vi "Read GUI Settings (SubVI).vi"(11 "File Path":path=path "C:/MWT/Config.ini") -> (3 "GUI Parameters":T1={"Image Width"=3072, "Image Height"=3072, "Pixel Intensity Low"=25, "Pixel Intensity High"=135, "Box Side Low"=6, "Box Side High"=200, "Box W+L Low"=12, "Box W+L High"=200, "Area Low"=12, "Area High"=200, "BG SUB TH"=200, "N Spine Points"=11.0, "Min Contour Points"=127, "Pixel Resolution (um/Pixel)"=40.69, "Gamma"=0.2} {"Gamma" format="%#_13g"; "Pixel Resolution (um/Pixel)" format="%#_13g"})   [LabVIEW 2020]
uses:
  Controls (HOST)/GUI Param.ctl
  Controls (HOST)/GUI Param List.ctl
  <vilib>/Utility/config.llb/Read Key (U32).vi
  <vilib>/Utility/config.llb/Write Key (U32).vi
  <vilib>/Utility/config.llb/Read Key (I32).vi
  <vilib>/Utility/config.llb/Write Key (I32).vi
  <vilib>/Utility/config.llb/Read Key (Double).vi
  <vilib>/Utility/config.llb/Write Key (Double).vi
  <vilib>/Utility/config.llb/NI_LVConfig.lvlib
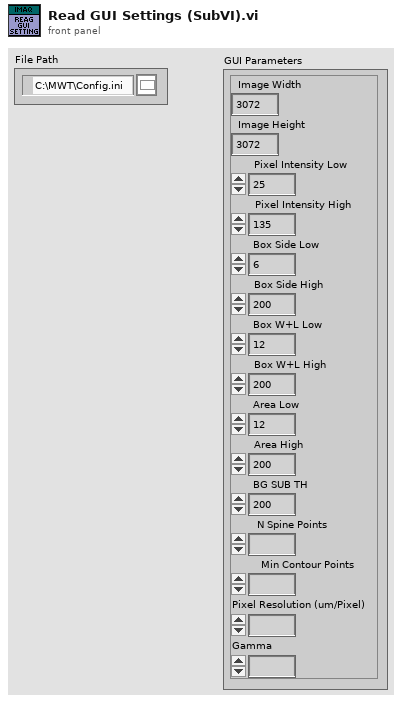
[diagram p1: front panel]
types:
  T1 = typedef "GUI Param.ctl" = cluster{"Image Width":u16, "Image Height":u16, "Pixel Intensity Low":u8, "Pixel Intensity High":u8, "Box Side Low":u32, "Box Side High":u32, "Box W+L Low":u32, "Box W+L High":u32, "Area Low":u32, "Area High":u32, "BG SUB TH":i16, "N Spine Points":fxp<+,8,8>, "Min Contour Points":u16, "Pixel Resolution (um/Pixel)":dbl, "Gamma":dbl}
  T2 = typedef "GUI Param List.ctl" = enum16{"None", "Image Height", "Image Width", "Pixel Intensity Low", "Pixel Intensity High", "Box Side Low", "Box Side High", "Box W+L Low", "Box W+L High", "Area Low", "Area High", "BG Sub Threshold", "N Spine Points", "Min Contour Points", "Pixel Resolution", "Gamma"}
  T3 = typedef "NI_LVConfig.lvlib/Config Data RefNum.ctl" = refnum<k1>
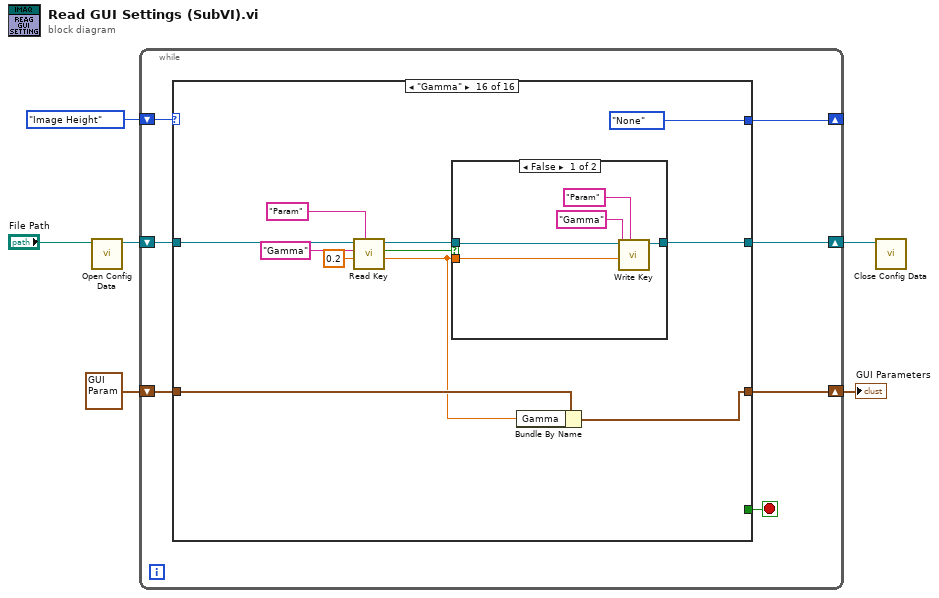
[diagram p0: block diagram]
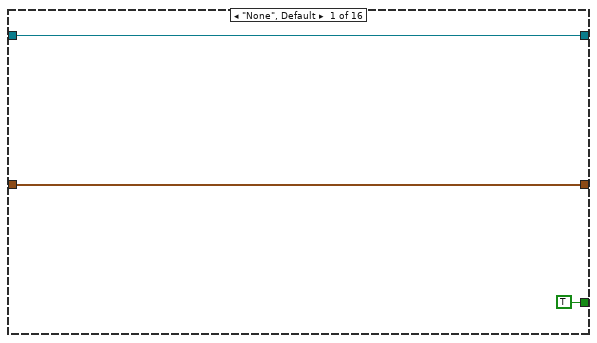
[diagram p2: hidden frame]
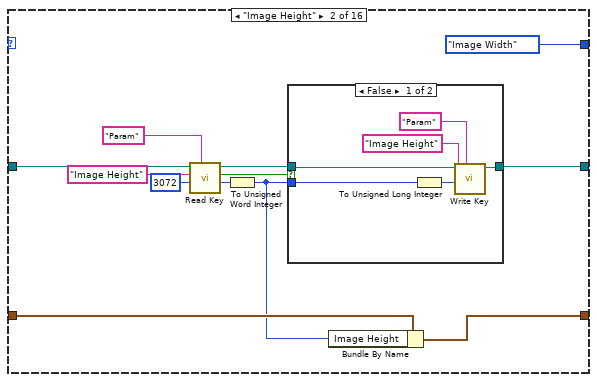
[diagram p3: hidden frame]
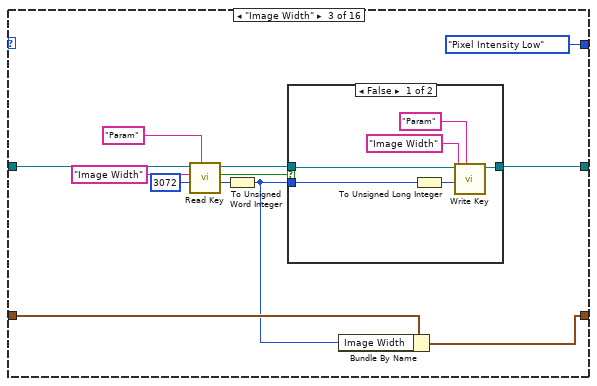
[diagram p5: hidden frame]
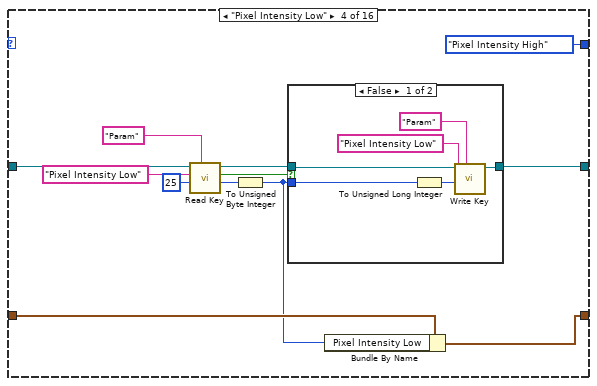
[diagram p7: hidden frame]
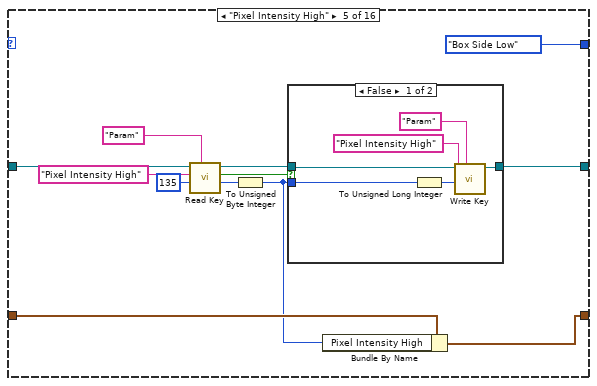
[diagram p9: hidden frame]
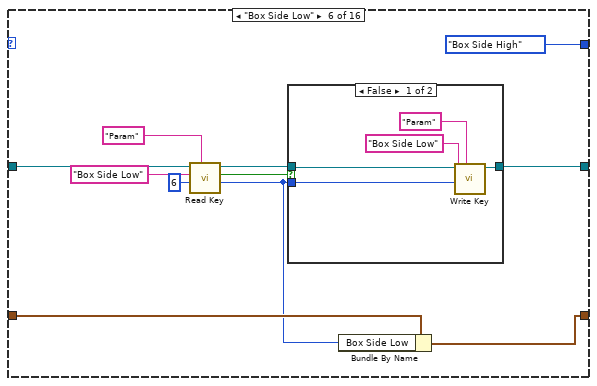
[diagram p11: hidden frame]
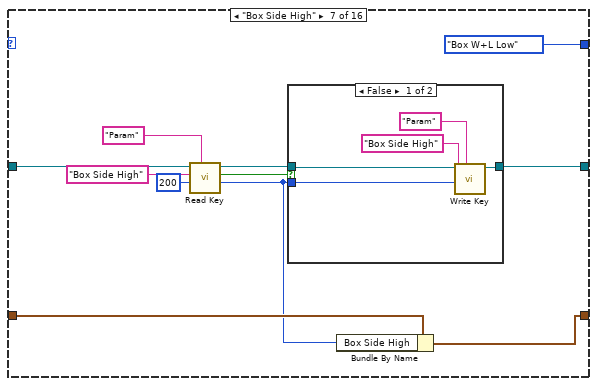
[diagram p13: hidden frame]
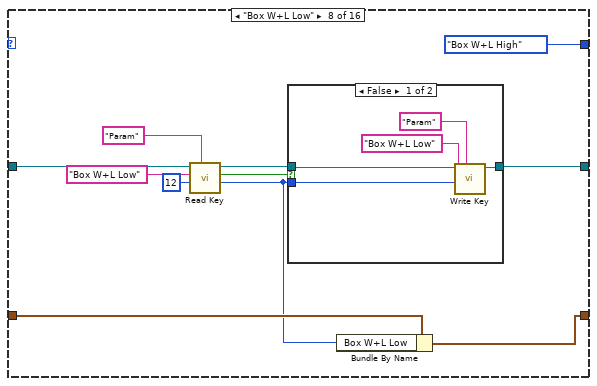
[diagram p15: hidden frame]
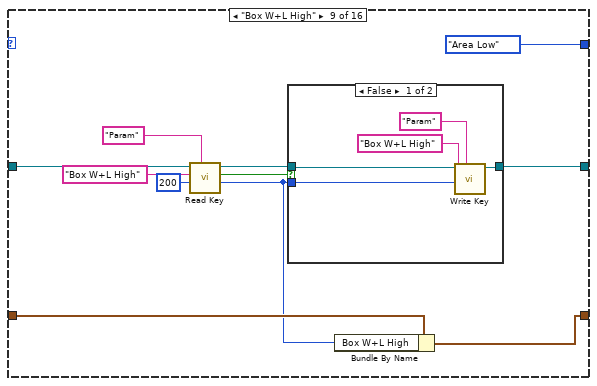
[diagram p17: hidden frame]
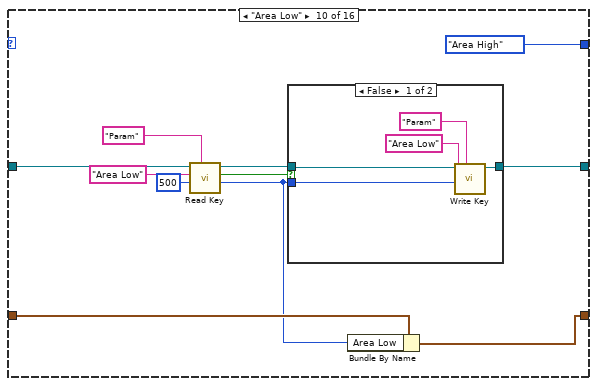
[diagram p19: hidden frame]
diagram:
  n1 = call <vilib>:"Open Config Data.vi"("configuration file path"="File Path") -> ("refnum"=w6:T3)  [unwired: 8 in, 2 out]
  n2 = while {
    shift-right: [w12] -> w4
    shift-left: w6 -> [w13]
    shift-right: [w9] -> _
    shift-left: GUI_Param_List."Image Height" -> [w11]
    shift-right: [w7] -> w1
    shift-left: T1 {"Image Width"=3072, "Image Height"=3072, "Pixel Intensity Low"=25, "Pixel Intensity High"=135, "Box Side Low"=6, "Box Side High"=200, "Box W+L Low"=12, "Box W+L High"=200, "Area Low"=12, "Area High"=200, "BG SUB TH"=200, "N Spine Points"=11.0, "Min Contour Points"=200, "Pixel Resolution (um/Pixel)"=40.69, "Gamma"=0.2} -> [w8]
    stop <- w10 stop-if-true
    n3 = case shown="\"Gamma\"" w11 {
      tunnel: w13 -> [w16 w24 w43 w63 w82 w100 w117 w134 w151 w168 w185 w203 w221 w239 w256 w273]
      tunnel: [w16 w21 w40 w60 w79 w97 w114 w131 w148 w165 w182 w200 w218 w236 w253 w270] -> w12
      tunnel: [TRUE _ _ _ _ _ _ _ _ _ _ _ _ _ _ _] -> w10
      tunnel: [_ GUI_Param_List."Image Width" GUI_Param_List."Pixel Intensity Low" GUI_Param_List."Pixel Intensity High" GUI_Param_List."Box Side Low" GUI_Param_List."Box Side High" GUI_Param_List."Box W+L Low" GUI_Param_List."Box W+L High" GUI_Param_List."Area Low" GUI_Param_List."Area High" GUI_Param_List."BG Sub Threshold" GUI_Param_List."N Spine Points" GUI_Param_List."Min Contour Points" GUI_Param_List."Pixel Resolution" GUI_Param_List."Gamma" GUI_Param_List."None"] -> w9
      tunnel: w8 -> [w14 w19 w38 w58 w77 w95 w112 w129 w146 w163 w180 w198 w216 w234 w251 w268]
      tunnel: [w14 w18 w37 w57 w76 w94 w111 w128 w145 w162 w179 w197 w215 w233 w250 w267] -> w7
      frame "None", Default {
      }
      frame "Image Height" {
        n4 = call-poly <vilib>:"Read Key.vi"("section"="Param", "default value"=u32 3072, "key"="Image Height" ("section"), "refnum"=w24) -> ("value"=w28:u32, "found?"=w23:bool, "refnum out"=w22:T3)  [unwired: 4 in, 1 out]
        n5 = To Unsigned Word Integer(number=w28) -> (unsigned 16bit integer=w17:u16)
        n6 = case shown="False" w23 {
          tunnel: w22 -> [w31 w35]
          tunnel: [w30 w35] -> w21
          tunnel: w17 -> [w29 _]
          frame False {
            n7 = To Unsigned Long Integer(number=w29) -> (unsigned 32bit integer=w33:u32)
            n8 = call-poly <vilib>:"Write Key.vi"("section"="Param", "value"=w33, "key"="Image Height" ("section"), "refnum"=w31) -> ("refnum out"=w30:T3)  [unwired: 5 in, 2 out]
          }
          frame True {
          }
        }
        n9 = Bundle By Name(cluster=w19, "Image Height"=w17) -> (w18:T1)
      }
      frame "Image Width" {
        n10 = call-poly <vilib>:"Read Key.vi"("section"="Param", "default value"=u32 3072, "key"="Image Width" ("section"), "refnum"=w43) -> ("value"=w47:u32, "found?"=w42:bool, "refnum out"=w41:T3)  [unwired: 4 in, 1 out]
        n11 = To Unsigned Word Integer(number=w47) -> (unsigned 16bit integer=w36:u16)
        n12 = case shown="False" w42 {
          tunnel: w41 -> [w50 w54]
          tunnel: [w49 w54] -> w40
          tunnel: w36 -> [w48 _]
          frame False {
            n13 = To Unsigned Long Integer(number=w48) -> (unsigned 32bit integer=w52:u32)
            n14 = call-poly <vilib>:"Write Key.vi"("section"="Param", "value"=w52, "key"="Image Width" ("section"), "refnum"=w50) -> ("refnum out"=w49:T3)  [unwired: 5 in, 2 out]
          }
          frame True {
          }
        }
        n15 = Bundle By Name(cluster=w38, "Image Width"=w36) -> (w37:T1)
      }
      frame "Pixel Intensity Low" {
        n16 = call-poly <vilib>:"Read Key.vi"("section"="Param", "default value"=u32 25, "key"="Pixel Intensity Low" ("section"), "refnum"=w63) -> ("value"=w56:u32, "found?"=w62:bool, "refnum out"=w61:T3)  [unwired: 4 in, 1 out]
        n17 = To Unsigned Byte Integer(number=w56) -> (unsigned 8bit integer=w55:u8)
        n18 = case shown="False" w62 {
          tunnel: w61 -> [w69 w73]
          tunnel: [w68 w73] -> w60
          tunnel: w55 -> [w67 _]
          frame False {
            n19 = To Unsigned Long Integer(number=w67) -> (unsigned 32bit integer=w71:u32)
            n20 = call-poly <vilib>:"Write Key.vi"("section"="Param", "value"=w71, "key"="Pixel Intensity Low" ("section"), "refnum"=w69) -> ("refnum out"=w68:T3)  [unwired: 5 in, 2 out]
          }
          frame True {
          }
        }
        n21 = Bundle By Name(cluster=w58, "Pixel Intensity Low"=w55) -> (w57:T1)
      }
      frame "Pixel Intensity High" {
        n22 = call-poly <vilib>:"Read Key.vi"("section"="Param", "default value"=u32 135, "key"="Pixel Intensity High" ("section"), "refnum"=w82) -> ("value"=w75:u32, "found?"=w81:bool, "refnum out"=w80:T3)  [unwired: 4 in, 1 out]
        n23 = To Unsigned Byte Integer(number=w75) -> (unsigned 8bit integer=w74:u8)
        n24 = case shown="False" w81 {
          tunnel: w80 -> [w88 w92]
          tunnel: [w87 w92] -> w79
          tunnel: w74 -> [w86 _]
          frame False {
            n25 = To Unsigned Long Integer(number=w86) -> (unsigned 32bit integer=w90:u32)
            n26 = call-poly <vilib>:"Write Key.vi"("section"="Param", "value"=w90, "key"="Pixel Intensity High" ("section"), "refnum"=w88) -> ("refnum out"=w87:T3)  [unwired: 5 in, 2 out]
          }
          frame True {
          }
        }
        n27 = Bundle By Name(cluster=w77, "Pixel Intensity High"=w74) -> (w76:T1)
      }
      frame "Box Side Low" {
        n28 = call-poly <vilib>:"Read Key.vi"("section"="Param", "default value"=u32 6, "key"="Box Side Low" ("section"), "refnum"=w100) -> ("value"=w93:u32, "found?"=w99:bool, "refnum out"=w98:T3)  [unwired: 4 in, 1 out]
        n29 = case shown="False" w99 {
          tunnel: w98 -> [w106 w109]
          tunnel: [w105 w109] -> w97
          tunnel: w93 -> [w104 _]
          frame False {
            n30 = call-poly <vilib>:"Write Key.vi"("section"="Param", "value"=w104, "key"="Box Side Low" ("section"), "refnum"=w106) -> ("refnum out"=w105:T3)  [unwired: 5 in, 2 out]
          }
          frame True {
          }
        }
        n31 = Bundle By Name(cluster=w95, "Box Side Low"=w93) -> (w94:T1)
      }
      frame "Box Side High" {
        n32 = call-poly <vilib>:"Read Key.vi"("section"="Param", "default value"=u32 200, "key"="Box Side High" ("section"), "refnum"=w117) -> ("value"=w110:u32, "found?"=w116:bool, "refnum out"=w115:T3)  [unwired: 4 in, 1 out]
        n33 = case shown="False" w116 {
          tunnel: w115 -> [w123 w126]
          tunnel: [w122 w126] -> w114
          tunnel: w110 -> [w121 _]
          frame False {
            n34 = call-poly <vilib>:"Write Key.vi"("section"="Param", "value"=w121, "key"="Box Side High" ("section"), "refnum"=w123) -> ("refnum out"=w122:T3)  [unwired: 5 in, 2 out]
          }
          frame True {
          }
        }
        n35 = Bundle By Name(cluster=w112, "Box Side High"=w110) -> (w111:T1)
      }
      frame "Box W+L Low" {
        n36 = call-poly <vilib>:"Read Key.vi"("section"="Param", "default value"=u32 12, "key"="Box W+L Low" ("section"), "refnum"=w134) -> ("value"=w127:u32, "found?"=w133:bool, "refnum out"=w132:T3)  [unwired: 4 in, 1 out]
        n37 = case shown="False" w133 {
          tunnel: w132 -> [w140 w143]
          tunnel: [w139 w143] -> w131
          tunnel: w127 -> [w138 _]
          frame False {
            n38 = call-poly <vilib>:"Write Key.vi"("section"="Param", "value"=w138, "key"="Box W+L Low" ("section"), "refnum"=w140) -> ("refnum out"=w139:T3)  [unwired: 5 in, 2 out]
          }
          frame True {
          }
        }
        n39 = Bundle By Name(cluster=w129, "Box W+L Low"=w127) -> (w128:T1)
      }
      frame "Box W+L High" {
        n40 = call-poly <vilib>:"Read Key.vi"("section"="Param", "default value"=u32 200, "key"="Box W+L High" ("section"), "refnum"=w151) -> ("value"=w144:u32, "found?"=w150:bool, "refnum out"=w149:T3)  [unwired: 4 in, 1 out]
        n41 = case shown="False" w150 {
          tunnel: w149 -> [w157 w160]
          tunnel: [w156 w160] -> w148
          tunnel: w144 -> [w155 _]
          frame False {
            n42 = call-poly <vilib>:"Write Key.vi"("section"="Param", "value"=w155, "key"="Box W+L High" ("section"), "refnum"=w157) -> ("refnum out"=w156:T3)  [unwired: 5 in, 2 out]
          }
          frame True {
          }
        }
        n43 = Bundle By Name(cluster=w146, "Box W+L High"=w144) -> (w145:T1)
      }
      frame "Area Low" {
        n44 = call-poly <vilib>:"Read Key.vi"("section"="Param", "default value"=u32 500, "key"="Area Low" ("section"), "refnum"=w168) -> ("value"=w161:u32, "found?"=w167:bool, "refnum out"=w166:T3)  [unwired: 4 in, 1 out]
        n45 = case shown="False" w167 {
          tunnel: w166 -> [w174 w177]
          tunnel: [w173 w177] -> w165
          tunnel: w161 -> [w172 _]
          frame False {
            n46 = call-poly <vilib>:"Write Key.vi"("section"="Param", "value"=w172, "key"="Area Low" ("section"), "refnum"=w174) -> ("refnum out"=w173:T3)  [unwired: 5 in, 2 out]
          }
          frame True {
          }
        }
        n47 = Bundle By Name(cluster=w163, "Area Low"=w161) -> (w162:T1)
      }
      frame "Area High" {
        n48 = call-poly <vilib>:"Read Key.vi"("section"="Param", "default value"=u32 3500, "key"="Area High" ("section"), "refnum"=w185) -> ("value"=w178:u32, "found?"=w184:bool, "refnum out"=w183:T3)  [unwired: 4 in, 1 out]
        n49 = case shown="False" w184 {
          tunnel: w183 -> [w191 w194]
          tunnel: [w190 w194] -> w182
          tunnel: w178 -> [w189 _]
          frame False {
            n50 = call-poly <vilib>:"Write Key.vi"("section"="Param", "value"=w189, "key"="Area High" ("section"), "refnum"=w191) -> ("refnum out"=w190:T3)  [unwired: 5 in, 2 out]
          }
          frame True {
          }
        }
        n51 = Bundle By Name(cluster=w180, "Area High"=w178) -> (w179:T1)
      }
      frame "BG Sub Threshold" {
        n52 = call-poly <vilib>:"Read Key.vi"("section"="Param", "default value"=10, "key"="BG SUB TH" ("section"), "refnum"=w203) -> ("value"=w196:i32, "found?"=w202:bool, "refnum out"=w201:T3)  [unwired: 4 in, 1 out]
        n53 = case shown="False" w202 {
          tunnel: w201 -> [w209 w212]
          tunnel: [w208 w212] -> w200
          tunnel: w196 -> [w207 _]
          frame False {
            n54 = call-poly <vilib>:"Write Key.vi"("section"="Param", "value"=w207, "key"="BG SUB TH" ("section"), "refnum"=w209) -> ("refnum out"=w208:T3)  [unwired: 5 in, 2 out]
          }
          frame True {
          }
        }
        n55 = To Word Integer(number=w196) -> (16bit integer=w195:i16)
        n56 = Bundle By Name(cluster=w198, "BG SUB TH"=w195) -> (w197:T1)
      }
      frame "N Spine Points" {
        n57 = call-poly <vilib>:"Read Key.vi"("section"="Param", "default value"=u32 11, "key"="N Spine Points" ("section"), "refnum"=w221) -> ("value"=w214:u32, "found?"=w220:bool, "refnum out"=w219:T3)  [unwired: 4 in, 1 out]
        n58 = case shown="False" w220 {
          tunnel: w219 -> [w227 w230]
          tunnel: [w226 w230] -> w218
          tunnel: w214 -> [w225 _]
          frame False {
            n59 = call-poly <vilib>:"Write Key.vi"("section"="Param", "value"=w225, "key"="N Spine Points" ("section"), "refnum"=w227) -> ("refnum out"=w226:T3)  [unwired: 5 in, 2 out]
          }
          frame True {
          }
        }
        n60 = To Fixed-Point(number=w214) -> (fixed-point=w213:fxp<+,8,8>)  [unwired: 1 in]
        n61 = Bundle By Name(cluster=w216, "N Spine Points"=w213) -> (w215:T1)
      }
      frame "Min Contour Points" {
        n62 = call-poly <vilib>:"Read Key.vi"("section"="Param", "default value"=u32 127, "key"="Min Contour Points" ("section"), "refnum"=w239) -> ("value"=w232:u32, "found?"=w238:bool, "refnum out"=w237:T3)  [unwired: 4 in, 1 out]
        n63 = case shown="False" w238 {
          tunnel: w237 -> [w245 w248]
          tunnel: [w244 w248] -> w236
          tunnel: w232 -> [w243 _]
          frame False {
            n64 = call-poly <vilib>:"Write Key.vi"("section"="Param", "value"=w243, "key"="Min Contour Points" ("section"), "refnum"=w245) -> ("refnum out"=w244:T3)  [unwired: 5 in, 2 out]
          }
          frame True {
          }
        }
        n65 = To Unsigned Word Integer(number=w232) -> (unsigned 16bit integer=w231:u16)
        n66 = Bundle By Name(cluster=w234, "Min Contour Points"=w231) -> (w233:T1)
      }
      frame "Pixel Resolution" {
        n67 = call-poly <vilib>:"Read Key.vi"("section"="Param", "default value"=40.69, "key"="Pixel Resolution" ("section"), "refnum"=w256) -> ("value"=w249:dbl, "found?"=w255:bool, "refnum out"=w254:T3)  [unwired: 4 in, 1 out]
        n68 = case shown="False" w255 {
          tunnel: w254 -> [w262 w265]
          tunnel: [w261 w265] -> w253
          tunnel: w249 -> [w260 _]
          frame False {
            n69 = call-poly <vilib>:"Write Key.vi"("section"="Param", "value"=w260, "key"="Pixel Resolution" ("section"), "refnum"=w262) -> ("refnum out"=w261:T3)  [unwired: 5 in, 2 out]
          }
          frame True {
          }
        }
        n70 = Bundle By Name(cluster=w251, "Pixel Resolution (um/Pixel)"=w249) -> (w250:T1)
      }
      frame "Gamma" {
        n71 = call-poly <vilib>:"Read Key.vi"("section"="Param", "default value"=0.2, "key"="Gamma" ("section"), "refnum"=w273) -> ("value"=w266:dbl, "found?"=w272:bool, "refnum out"=w271:T3)  [unwired: 4 in, 1 out]
        n72 = case shown="False" w272 {
          tunnel: w271 -> [w279 w282]
          tunnel: [w278 w282] -> w270
          tunnel: w266 -> [w277 _]
          frame False {
            n73 = call-poly <vilib>:"Write Key.vi"("section"="Param", "value"=w277, "key"="Gamma" ("section"), "refnum"=w279) -> ("refnum out"=w278:T3)  [unwired: 5 in, 2 out]
          }
          frame True {
          }
        }
        n74 = Bundle By Name(cluster=w268, "Gamma"=w266) -> (w267:T1)
      }
    }
  }
  "GUI Parameters" <- w1
  n75 = call <vilib>:"Close Config Data.vi"("refnum"=w4) -> ()  [unwired: 9 in, 2 out]
